vi "DistillTitle.vi"(7 "Plot Summary in":string[][](array[string]), 8 "Show Channels with range of Values?":bool, 10 "Indices to include in Page Title":i32[](array[numeric]), 11 "String in":string) -> (3 "String out":string, 4 "AvailableVariables":string[](array[string]))   [LabVIEW 2014]
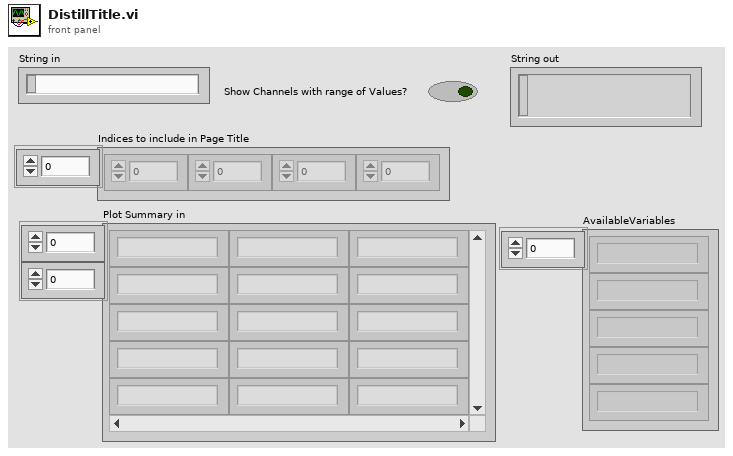
[diagram p1: front panel]
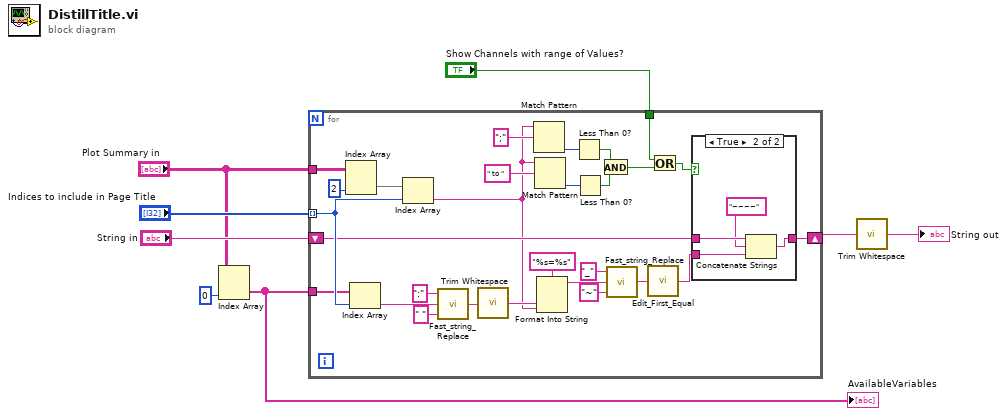
[diagram p0: block diagram]
diagram:
  n1 = Index Array(array="Plot Summary in", index (col)=0 ("disabled index (col)")) -> (element=w5:string[])  [unwired: 1 in]
  "AvailableVariables" <- w5
  n2 = for {
    tunnel: "Indices to include in Page Title" -> [w35] mode=indexing
    tunnel: "Plot Summary in" -> [w36]
    shift-right: [w26] -> w6
    shift-left: "String in" -> [w27]
    tunnel: w5 -> [w24]
    tunnel: "Show Channels with range of Values?" -> [w9]
    n3 = Index Array(array=w36, index (col)=2 ("index (row)")) -> (element=w34:string[])  [unwired: 1 in]
    n4 = Index Array(array=w24, index=w35) -> (element=w30:string)
    n5 = Index Array(array=w34, index=w35) -> (element=w21:string)
    n6 = call "Fast_string_Replace.vi"("Replace match with:"=" ", "Input String"=w30, "regular expression"=":") -> ("Output String"=w29:string)  [unwired: 2 out]
    n7 = call <vilib>:"Trim Whitespace.vi"("string"=w29) -> ("trimmed string"=w28:string)  [unwired: 1 in]
    n8 = Match Pattern(string=w21, regular expression=";") -> (offset past match=w17:i32)  [unwired: 4 out]
    n9 = Match Pattern(string=w21, regular expression=" to ") -> (offset past match=w18:i32)  [unwired: 4 out]
    n10 = Format Into String(format string="%s=%s", w28, w21) -> (resulting string=w14:string)  [unwired: 2 in, 1 out]
    n11 = Less Than 0?(x=w17) -> (x < 0?=w19:bool)
    n12 = Less Than 0?(x=w18) -> (x < 0?=w20:bool)
    n13 = And(x=w19, y=w20) -> (x .and. y?=w10:bool)
    n14 = call "Fast_string_Replace.vi"("Replace match with:"="~", "Input String"=w14, "regular expression"="_") -> ("Output String"=w13:string)  [unwired: 2 out]
    n15 = call "Edit_First_Equal.vi"("String in"=w13) -> ("String out"=w12:string)
    n16 = Or(x=w9, y=w10) -> (x .or. y?=w11:bool)
    n17 = case shown="True" w11 {
      tunnel: w27 -> [w37 w41]
      tunnel: [w37 w40] -> w26
      tunnel: w12 -> [_ w39]
      frame False {
      }
      frame True {
        n18 = Concatenate Strings(w41, "~~~~" ("string"), w39) -> (w40:string)
      }
    }
  }
  n19 = call <vilib>:"Trim Whitespace.vi"("string"=w6) -> ("trimmed string"=→"String out":string)  [unwired: 1 in]
